vi "XLP80_CAN_DemaskAndMask.vi"(7 "Function":string, 8 "err in":errorcluster, 11 "Variant":variant) -> (0 "error out":errorcluster, 3 "CANData Write":T1[](array[typedef]) {"ID" format="%.0x"})   [LabVIEW 2021]
uses:
  <userlib>/PCAN Basic/Controls/CAN MSG Cluster.ctl
  <vilib>/nican/nican.llb/ncNetAttr.ctl
  <vilib>/nican/nicantsk.llb/CAN Interface.ctl
  <vilib>/nican/nicantsk.llb/CAN Mode.ctl
  <vilib>/nican/nican.llb/CanFrameTimed.ctl
  XLP80_FGlob/1886_FGlob_TDefs_Enum_FGlobItems.ctl
  XLP80_Globals/Globals_Settings_XLP80.vi
  XLP80_Globals/XLP80_CAN_Globals.vi
  <vilib>/nican/nicantsk.llb/CAN Set Interface Virtual Bus Timing.vi
  XLP80_Globals/XLP80_Globals_Action.vi
  XLP80_Globals/XLP80_Globals_Status.vi
  <vilib>/nican/nicantsk.llb/CAN Write Multi Chan Single Samp 1D Dbl.vi
  <vilib>/nican/nicantsk.llb/CAN Read Multi Chan Single Samp 1D Dbl.vi
  <userlib>/PCAN Basic/PCANBasic.lvlib
panel:
  out "x+y":i32
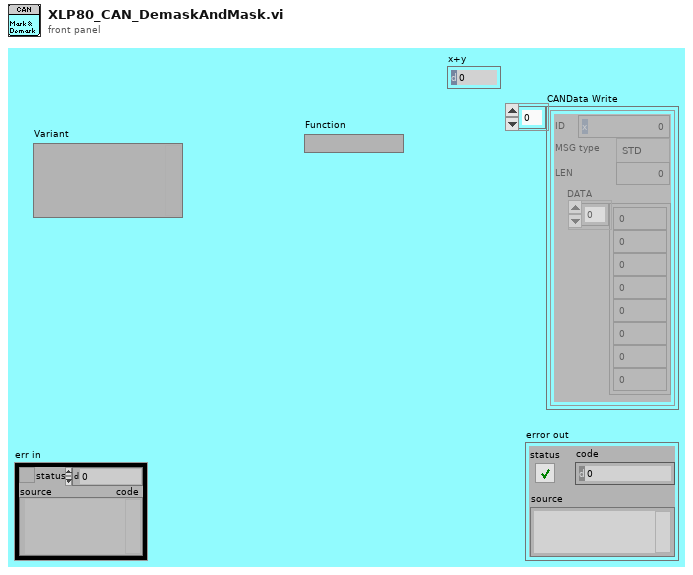
[diagram p1: front panel]
types:
  T1 = typedef "PCANBasic.lvlib/CAN MSG Cluster.ctl" = cluster{"ID":u32, "MSG type":enum8{"STD", "RTR", "XTD", "XTD RTR", "STATUS"}, "LEN":i8, "DATA":u8[]}
  T2 = cluster{"CAN DBC":path, "ReadSignal Name":string[], "WriteSignal Name":string[]}
  T3 = typedef "ncNetAttr.ctl" = cluster{"Start On Open":enum32{"FALSE", "TRUE"}, "Baud Rate":u32, "Read Queue Length":u32, "Write Queue Length":u32, "Standard Comparator":u32, "Standard Mask":u32, "Extended Comparator":u32, "Extended Mask":u32}
  T4 = typedef "1886_FGlob_TDefs_Enum_FGlobItems.ctl" = enum16{"Put one", "Put all", "Recall one", "Recall all"}
  T5 = typedef "CanFrameTimed.ctl" = cluster{"Timestamp":dbl, "ArbitrationId":u32, "IsRemote":u8, "DataLength":u8, "Data":u8[]}
  T6 = typedef "CAN Mode.ctl" = u16
  T7 = typedef "CAN Interface.ctl" = u16
  T8 = typedef "xobjhandle.ctl" = u32
  T9 = typedef "CAN Task Reference.ctl" = u32
  T10 = typedef "XLP80_Action_TDefEnumControl.ctl" = enum16{"Testmode_A", "Testmode_B"}
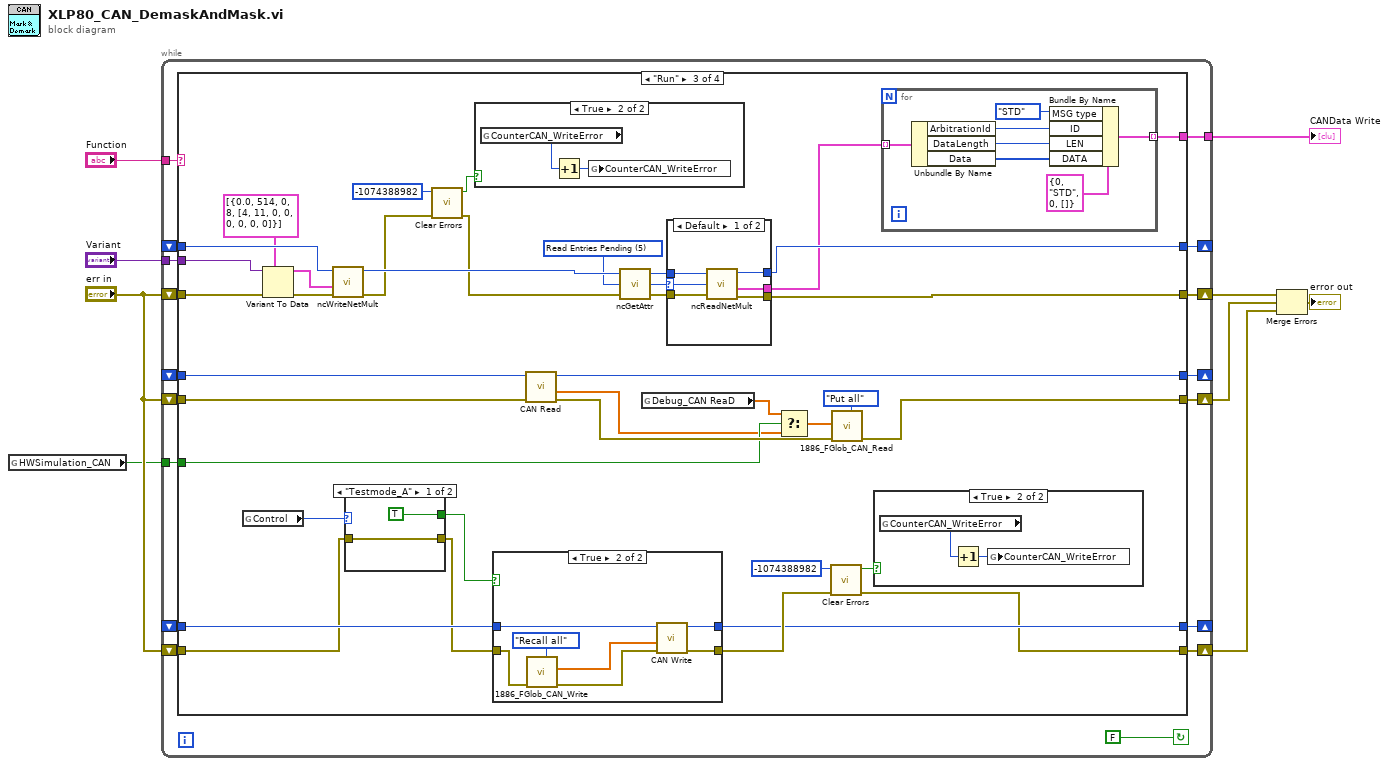
[diagram p0: block diagram]
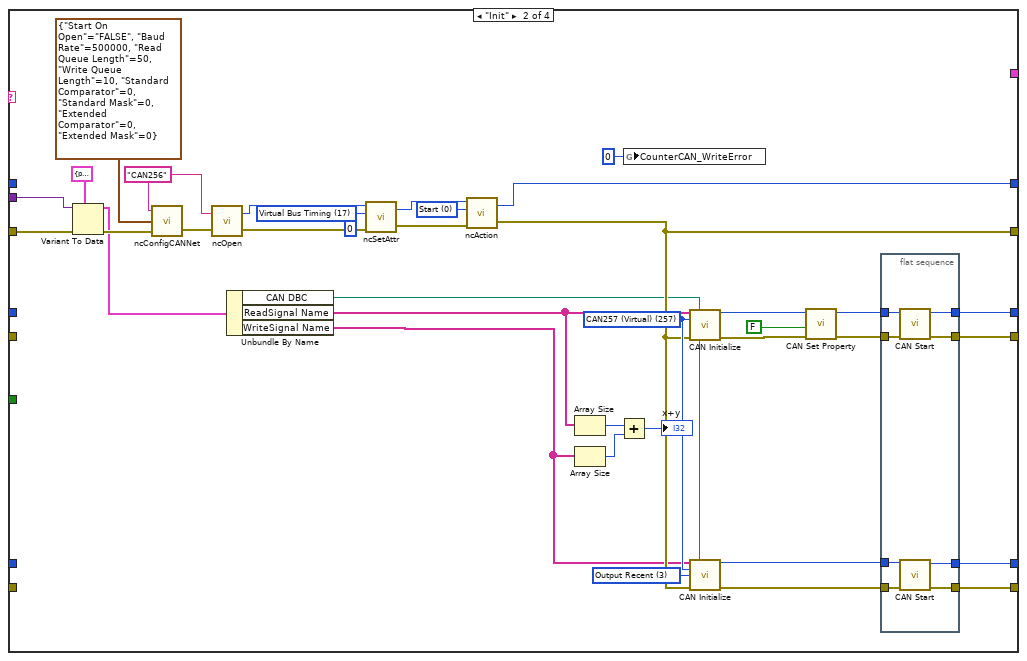
[diagram p3: hidden frame]
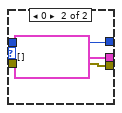
[diagram p4: hidden frame]
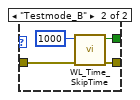
[diagram p6: hidden frame]
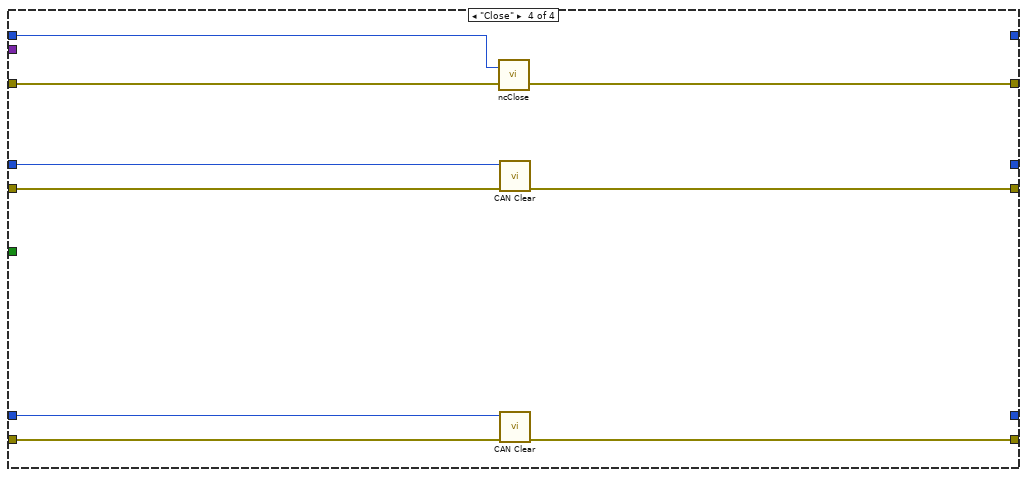
[diagram p9: hidden frame]
diagram:
  n1 = global read "Globals_Settings_XLP80.vi" "HWSimulation_CAN"() -> (w1:bool)
  n2 = while {
    shift-right: [w13] -> _
    shift-left: _ -> [w23]
    shift-right: [w16] -> w5
    shift-left: "err in" -> [w22]
    shift-right: [w24] -> _
    shift-left: _ -> [w26]
    shift-right: [w15] -> w6
    shift-left: "err in" -> [w25]
    shift-right: [w19] -> w7
    shift-left: "err in" -> [w21]
    shift-right: [w18] -> _
    shift-left: _ -> [w20]
    tunnel: "Function" -> [w14]
    tunnel: "Variant" -> [w12]
    tunnel: [w11] -> w2
    tunnel: w1 -> [w10]
    stop <- FALSE continue-if-true
    n3 = case shown="\"Run\"" w14 {
      tunnel: w26 -> [w30 _ w116 w156]
      tunnel: w25 -> [w29 _ w115 w157]
      tunnel: [w30 w47 w114 _] -> w24
      tunnel: w23 -> [w32 _ w112 w158]
      tunnel: w22 -> [w31 w44 w111 w160]
      tunnel: w21 -> [w27 _ w84 w154]
      tunnel: w20 -> [w28 _ w110 w155]
      tunnel: [w27 w46 w93 w153] -> w19
      tunnel: [w28 w45 w108 _] -> w18
      tunnel: [w31 w49 w106 w159] -> w16
      tunnel: [w29 w48 w105 w152] -> w15
      tunnel: [w32 w59 w104 _] -> w13
      tunnel: w12 -> [_ w42 w102 _]
      tunnel: [_ _ w99 _] -> w11
      tunnel: w10 -> [_ _ w97 _]
      frame Default {
      }
      frame "Init" {
        w58 = T6 3 items=["Input", "Output", "Timestamped Input", "Output Recent"] ("mode")
        w55 = T7 257 items=["CAN0"=0, "CAN1"=1, "CAN2"=2, "CAN3"=3, "CAN4"=4, "CAN5"=5, "CAN6"=6, "CAN7"=7, "CAN8"=8, "CAN9"=9, "CAN10"=10, "CAN11"=11, "CAN12"=12, "CAN13"=13, "CAN14"=14, "CAN15"=15, "CAN16"=16, "CAN17"=17, "CAN18"=18, "CAN19"=19, "CAN20"=20, "CAN21"=21, "CAN22"=22, "CAN23"=23, "CAN24"=24, "CAN25"=25, "CAN26"=26, "CAN27"=27, "CAN28"=28, "CAN29"=29, "CAN30"=30, "CAN31"=31, "CAN32"=32, "CAN33"=33, "CAN34"=34, "CAN35"=35, "CAN36"=36, "CAN37"=37, "CAN38"=38, "CAN39"=39, "CAN40"=40, "CAN41"=41, "CAN42"=42, "CAN43"=43, "CAN44"=44, "CAN45"=45, "CAN46"=46, "CAN47"=47, "CAN48"=48, "CAN49"=49, "CAN50"=50, "CAN51"=51, "CAN52"=52, "CAN53"=53, "CAN54"=54, "CAN55"=55, "CAN56"=56, "CAN57"=57, "CAN58"=58, "CAN59"=59, "CAN60"=60, "CAN61"=61, "CAN62"=62, "CAN63"=63, "MAX default"=64, "CAN256 (Virtual)"=256, "CAN257 (Virtual)"=257] ("interface")
        w68 = "CAN256" ("CAN")
        w66 = u32 0 items=["Start", "Stop", "Reset", "Output on RTSI line"] ("Opcode")
        w62 = u32 17 items=["ReadMult Size for Notification", "User RTSI Frame", "Log Comm Warnings", "Listen Only?", "Self Reception?", "Single Shot Transmit?", "Series 2 Filter Mode", "Series 2 Mask", "Series 2 Comparator", "Transceiver Type", "Transceiver Mode", "Transceiver External Outputs", "(reserved)", "Transmit Mode", "Log Start Trigger?", "Timestamp Format", "Master Timebase Rate", "Virtual Bus Timing", "Timeline Recovery", "Log Bus Error?", "Log Transceiver Fault?", "Termination", "LIN Sleep", "LIN Checksum Type", "LIN Response Timeout", "LIN Enable DLC Check", "LIN Log Wakeup", "Baud Rate"] ("AttrId")
        n4 = Variant To Data(error in=w44, type=T2 {"CAN DBC"=path "", "ReadSignal Name"=[], "WriteSignal Name"=[]} ("output cluster"), Variant=w42) -> (data=w41:T2, error out=w43:errorcluster)
        n5 = call <vilib>:"ncConfigCANNet.vi"("Error in"=w43, "CAN Network Interface Config"=T3 {"Start On Open"=enum."FALSE", "Baud Rate"=500000, "Read Queue Length"=50, "Write Queue Length"=10, "Standard Comparator"=0, "Standard Mask"=0, "Extended Comparator"=0, "Extended Mask"=0}, "ObjName"=w68) -> ("Error out"=w69:errorcluster)  [unwired: 2 in]
        n6 = call <vilib>:"ncOpen.vi"("Error in"=w69, "ObjName"=w68) -> ("Error out"=w64:errorcluster, "ObjHandle out"=w61:T8)
        n7 = Unbundle By Name(w41) -> ("CAN DBC"=w40:path, "ReadSignal Name"=w38:string[], "WriteSignal Name"=w34:string[])
        n8 = call <vilib>:"ncSetAttr.vi"("Error in"=w64, "AttrValue"=u32 0, "AttrId"=w62, "ObjHandle in"=w61) -> ("Error out"=w65:errorcluster, "ObjHandle out"=w67:T8)
        n9 = call <vilib>:"ncAction.vi"("Error in"=w65, "Opcode"=w66, "ObjHandle in"=w67) -> ("Error out"=w49:errorcluster, "ObjHandle out"=w59:T8)  [unwired: 1 in]
        n10 = Array Size(array=w38) -> (size(s)=w37:i32)
        n11 = Array Size(array=w34) -> (size(s)=w36:i32)
        n12 = Add(x=w37, y=w36) -> (x+y=→"x+y":i32)
        n13 = global write "XLP80_CAN_Globals.vi" "CounterCAN_WriteError"(0 ("CounterCAN_WriteError")) -> ()
        n14 = call <vilib>:"CAN Initialize.vi"("channel list"=w38, "filepath"=w40, "interface"=w55, "error in (no error)"=w49) -> ("task reference out"=w50:T9, "error out"=w52:errorcluster)  [unwired: 10 in]
        n15 = call <vilib>:"CAN Initialize.vi"("channel list"=w34, "filepath"=w40, "interface"=w55, "mode"=w58, "error in (no error)"=w49) -> ("task reference out"=w57:T9, "error out"=w56:errorcluster)  [unwired: 9 in]
        n16 = call-poly <vilib>:"CAN Set Property.vi"("error in (no error)"=w52, "virtual bus timing?"=FALSE, "task reference in"=w50) -> ("error out"=w53:errorcluster, "task reference out"=w54:T9)  [unwired: 7 in]
        n17 = flat-sequence {
          tunnel: w53 -> [w77]
          tunnel: [w76] -> w47
          tunnel: [w75] -> w48
          tunnel: w54 -> [w74]
          tunnel: w56 -> [w73]
          tunnel: w57 -> [w72]
          tunnel: [w71] -> w46
          tunnel: [w70] -> w45
          frame #0 {
            n18 = call <vilib>:"CAN Start.vi"("error in (no error)"=w77, "task reference"=w74) -> ("error out"=w75:errorcluster, "task reference out"=w76:T9)  [unwired: 8 in]
            n19 = call <vilib>:"CAN Start.vi"("error in (no error)"=w73, "task reference"=w72) -> ("error out"=w71:errorcluster, "task reference out"=w70:T9)  [unwired: 8 in]
          }
        }
      }
      frame "Run" {
        w82 = u32 5 items=["(reserved)", "Protocol Version", "Software Version", "Object State", "(reserved)", "Read Entries Pending", "Write Entries Pending", "ReadMult Size for Notification", "Listen Only?", "Self Reception?", "Transmit Error Counter", "Receive Error Counter", "Single Shot Transmit?", "Series 2 Filter Mode", "Series 2 Mask", "Series 2 Comparator", "Serial Number", "Form Factor", "Series", "Transceiver Type", "Interface Number", "Series 2 Error/Arb Capture", "Transceiver Mode", "Transceiver External Outputs", "Transceiver External Inputs", "Start Trigger Behavior", "Log Comm Warnings", "User RTSI Frame", "Transmit Mode", "Log Start Trigger?", "Timestamp Format", "Master Timebase Rate", "Virtual Bus Timing", "Write Entries Free", "Timeline Recovery", "Log Bus Errors", "Log Transceiver Faults", "Termination", "LIN Sleep", "LIN Checksum Type", "LIN Response Timeout", "LIN Enable DLC Check", "LIN Log Wakeup", "Baud Rate"] ("AttrId")
        n20 = global read "XLP80_Globals_Status.vi" "Control"() -> (w85:T10)
        n21 = Variant To Data(error in=w111, type=T5[] [{"Timestamp"=0.0, "ArbitrationId"=514, "IsRemote"=0, "DataLength"=8, "Data"=[4, 11, 0, 0, 0, 0, 0, 0]}] ("Data"), Variant=w102) -> (data=w86:T5[], error out=w103:errorcluster)
        n22 = call <vilib>:"ncWriteNetMult.vi"("Error in"=w103, "Data"=w86, "ObjHandle in"=w112) -> ("Error out"=w88:errorcluster, "ObjHandle out"=w107:T8)  [unwired: 7 in]
        n23 = case shown="\"Testmode_A\"" w85 {
          tunnel: w84 -> [w136 w140]
          tunnel: [w136 w139] -> w83
          tunnel: [TRUE ("Run") w137] -> w78
          frame "Testmode_A" {
          }
          frame "Testmode_B" {
            n24 = call "WL_Time_SkipTime.vi"("err in"=w140, "SkipTime[ms]"=u32 1000) -> ("err out"=w139:errorcluster, "Run"=w137:bool)  [unwired: 8 in]
          }
        }
        n25 = call <vilib>:"Clear Errors.vi"("error in (no error)"=w88, "specific error code to clear (0: all)"=-1074388982) -> ("error out"=w87:errorcluster, "specific error cleared?"=w90:bool)  [unwired: 4 in]
        n26 = case shown="True" w90 {
          frame False {
          }
          frame True {
            n27 = global read "XLP80_CAN_Globals.vi" "CounterCAN_WriteError"() -> (w141:i32)
            n28 = Increment(x=w141) -> (x+1=w142:i32)
            n29 = global write "XLP80_CAN_Globals.vi" "CounterCAN_WriteError"(w142) -> ()
          }
        }
        n30 = case shown="True" w78 {
          tunnel: w110 -> [w127 w134]
          tunnel: [w126 w133] -> w109
          tunnel: [w127 w132] -> w108
          tunnel: w83 -> [w126 w128]
          frame False {
          }
          frame True {
            n31 = call "1886_FGlob_CAN_Write.vi"("Function (Recall One)"=1886_FGlob_TDefs_Enum_FGlobItems."Recall all", "err in"=w128) -> ("err out"=w131:errorcluster, "AO Values OUT"=w129:dbl[])  [unwired: 7 in, 1 out]
            n32 = call-poly <vilib>:"CAN Write.vi"("error in (no error)"=w131, "multi-chan single-samp 1D dbl"=w129, "task reference in"=w134) -> ("error out"=w133:errorcluster, "task reference out"=w132:T9)  [unwired: 7 in]
          }
        }
        n33 = call-poly <vilib>:"CAN Read.vi"("error in (no error)"=w115, "task reference in"=w116) -> ("error out"=w113:errorcluster, "multi-chan single-samp 1D dbl"=w96:dbl[], "task reference out"=w114:T9)  [unwired: 6 in, 1 out]
        n34 = call <vilib>:"ncGetAttr.vi"("Error in"=w87, "AttrId"=w82, "ObjHandle in"=w107) -> ("Error out"=w81:errorcluster, "AttrValue"=w79:u32, "ObjHandle out"=w80:T8)
        n35 = global read "XLP80_Globals_Action.vi" "Debug_CAN ReaD"() -> (w95:dbl[])
        n36 = case shown="Default" w79 {
          selector: w79 -> [w117 _]
          tunnel: [w122 w124] -> w106
          tunnel: [w121 w125] -> w104
          tunnel: [w120 T5[] [] ("Data")] -> w100
          tunnel: w80 -> [w119 w125]
          tunnel: w81 -> [w118 w124]
          frame Default {
            n37 = call <vilib>:"ncReadNetMult.vi"("ObjHandle in"=w119, "Requested Number of Frames"=w117, "Error in"=w118) -> ("ObjHandle out"=w121:T8, "Data"=w120:T5[], "Error out"=w122:errorcluster)  [unwired: 1 out]
          }
          frame 0 {
          }
        }
        n38 = Select(t=w95, s=w97, f=w96) -> (s? t:f=w94:dbl[])
        n39 = call <vilib>:"Clear Errors.vi"("error in (no error)"=w109, "specific error code to clear (0: all)"=-1074388982) -> ("error out"=w93:errorcluster, "specific error cleared?"=w91:bool)  [unwired: 4 in]
        n40 = call "1886_FGlob_CAN_Read.vi"("Function (Recall One)"=1886_FGlob_TDefs_Enum_FGlobItems."Put all", "err in"=w113, "AI Values IN"=w94) -> ("err out"=w105:errorcluster)  [unwired: 6 in, 2 out]
        n41 = case shown="True" w91 {
          frame False {
          }
          frame True {
            n42 = global read "XLP80_CAN_Globals.vi" "CounterCAN_WriteError"() -> (w143:i32)
            n43 = Increment(x=w143) -> (x+1=w144:i32)
            n44 = global write "XLP80_CAN_Globals.vi" "CounterCAN_WriteError"(w144) -> ()
          }
        }
        n45 = for {
          tunnel: w100 -> [w151] mode=indexing
          tunnel: [w145] -> w99 mode=indexing
          n46 = Unbundle By Name(w151) -> ("ArbitrationId"=w149:u32, "DataLength"=w147:u8, "Data"=w146:u8[])
          n47 = Bundle By Name(cluster=T1 {"ID"=0, "MSG type"=enum."STD", "LEN"=0, "DATA"=[]} ("CAN_Message out"), "MSG type"=enum8{"STD", "RTR", "XTD", "XTD RTR", "STATUS"}."STD", "ID"=w149, "LEN"=w147, "DATA"=w146) -> (w145:T1)
        }
      }
      frame "Close" {
        n48 = call <vilib>:"ncClose.vi"("Error in"=w160, "ObjHandle in"=w158) -> ("Error out"=w159:errorcluster)  [unwired: 1 in]
        n49 = call <vilib>:"CAN Clear.vi"("error in (no error)"=w157, "task reference in"=w156) -> ("error out"=w152:errorcluster)  [unwired: 9 in]
        n50 = call <vilib>:"CAN Clear.vi"("error in (no error)"=w154, "task reference in"=w155) -> ("error out"=w153:errorcluster)  [unwired: 9 in]
      }
    }
  }
  "CANData Write" <- w2
  n51 = Merge Errors(w5, w6, w7) -> (→"error out":errorcluster)
